vi "Set Read Access.vi"(8 "error in (no error)":errorcluster, 10 "Read Access":enum8{"Allowed", "Required", "None"}(ring), 11 "abs_SharedVar_Bool in":refnum<class "conc_SharedVar_SGL.lvclass">) -> (0 "error out":errorcluster, 3 "abs_SharedVar_Bool out":refnum<class "conc_SharedVar_SGL.lvclass">)   [LabVIEW 2021, in "conc_SharedVar_SGL.lvclass"]
uses:
  conc_SharedVar_SGL.lvclass
  conc_SharedVar_SGL.lvclass/conc_SharedVar_SGL.ctl
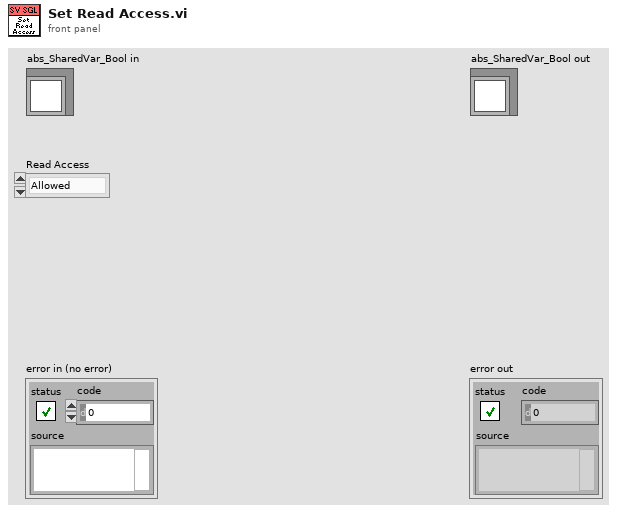
[diagram p1: front panel]
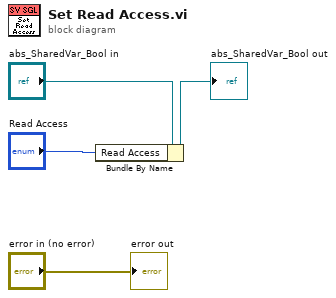
[diagram p0: block diagram]
diagram:
  n1 = Bundle By Name(cluster="abs_SharedVar_Bool in", "Read Access"="Read Access") -> (→"abs_SharedVar_Bool out":refnum<class "conc_SharedVar_SGL.lvclass">)
  "error out" <- "error in (no error)"
